vi "HUR.vi"(4 "Delta T (K)":dbl, 6 "Heating Power (W)":dbl, 7 "Time":dbl, 9 "Cp (J/kgK)":dbl, 10 "Mass Flow (kg/s)":dbl, 11 "Hot Mass (kg)":dbl) -> (2 "Cooling Power (W)":dbl, 3 "HUR (K)":dbl)   [LabVIEW 2019]
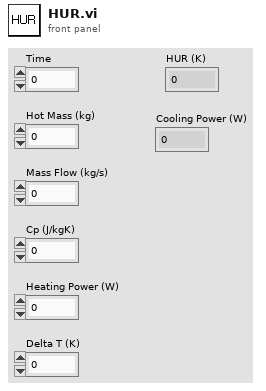
[diagram p1: front panel]
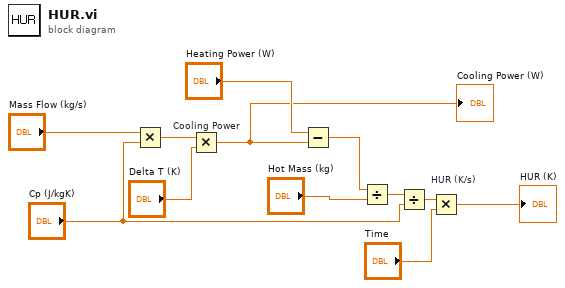
[diagram p0: block diagram]
diagram:
  n1 = Multiply(x="Mass Flow (kg/s)", y="Cp (J/kgK)") -> (x*y=w3:dbl)
  n2 = Multiply "Cooling Power"(x=w3, y="Delta T (K)") -> (x*y=w1:dbl)
  "Cooling Power (W)" <- w1
  n3 = Subtract(x="Heating Power (W)", y=w1) -> (x-y=w6:dbl)
  n4 = Divide(x=w6, y="Hot Mass (kg)") -> (x/y=w8:dbl)
  n5 = Divide(x=w8, y="Cp (J/kgK)") -> (x/y=w10:dbl)
  n6 = Multiply "HUR (K/s)"(x=w10, y="Time") -> (x*y=→"HUR (K)":dbl)
